vi "load_front_panel.vi"(4 "error in (no error)":errorcluster, 6 "VIpath":path, 7 "Sub Panel in":refnum<vi>) -> (0 "error out":errorcluster, 2 "front panel VI Refnum":refnum<vi>, 3 "Sub Panel out":refnum<vi>)   [LabVIEW 2010]
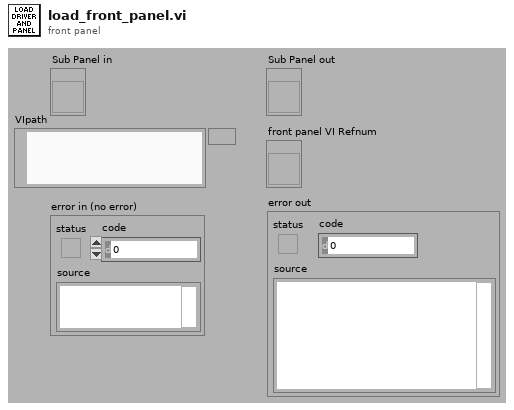
[diagram p1: front panel]
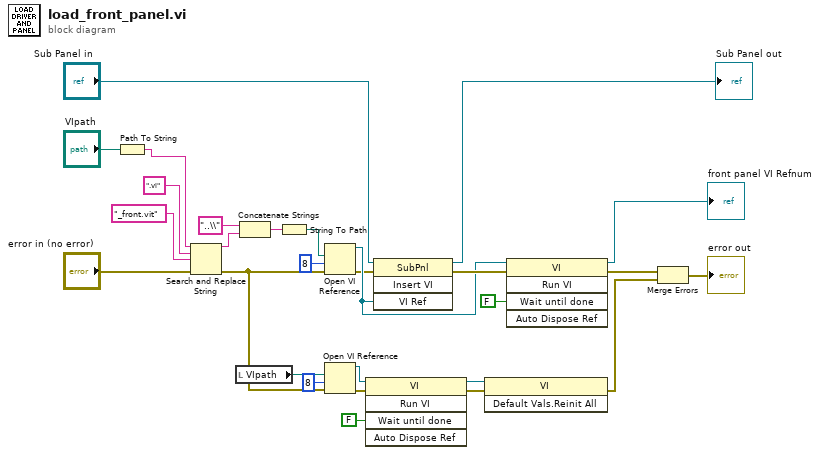
[diagram p0: block diagram]
diagram:
  n1 = Path To String(path="VIpath") -> (string=w14:string)
  n2 = Search and Replace String(input string=w14, search string=".vi", replace string="_front.vit" ("replace string (\"\")"), error in="error in (no error)") -> (result string=w16:string, error out=w1:errorcluster)  [unwired: 4 in, 2 out]
  n3 = local read "VIpath"() -> (w11:path)
  n4 = Concatenate Strings("..\\" ("string"), w16) -> (w13:string)
  n5 = String To Path(string=w13) -> (path=w12:path)
  n6 = Open VI Reference(vi path=w12, options=8, error in (no error)=w1) -> (vi reference=w26:refnum<vi>, error out=w23:errorcluster)  [unwired: 3 in]
  n7 = Open VI Reference(vi path=w11, options=8, error in (no error)=w1) -> (vi reference=w7:refnum<vi>, error out=w9:errorcluster)  [unwired: 3 in]
  n8 = invoke class="VI" method="Run VI"(reference=w7, error in=w9, "Wait until done"=FALSE ("Wait Until Done")) -> (reference out=w6:refnum<vi>, error out=w5:errorcluster)  [unwired: 2 in, 3 out]
  n9 = invoke class="SubPnl" method="Insert VI"(reference="Sub Panel in", error in=w23, "VI Ref"=w26) -> (reference out=→"Sub Panel out":refnum<vi>, error out=w27:errorcluster)  [unwired: 1 in, 2 out]
  n10 = invoke class="VI" method="Default Vals.Reinit All"(reference=w6, error in=w5) -> (error out=w3:errorcluster)  [unwired: 1 in, 2 out]
  n11 = invoke class="VI" method="Run VI"(reference=w26, error in=w27, "Wait until done"=FALSE ("Wait Until Done")) -> (reference out=→"front panel VI Refnum":refnum<vi>, error out=w4:errorcluster)  [unwired: 2 in, 3 out]
  n12 = Merge Errors(w4, w3) -> (→"error out":errorcluster)
